vi "SW_Generate_SubCondition_text.vi"(8 "error in (no error)":errorcluster, 11 "Condition":T1 {"Response"."TTL pulse length, ms" min=0.0 max=10000.0 step=10.0 format="%0.0g"; "Specifier(s)"."Validity criteria(s)"."Validity value" min=0.0 step=0.1 format="%.2g"; "Specifier(s)"."Value" step=1.0 format="%#.2g"}) -> (0 "error out":errorcluster, 3 "SubCondition text":string[](array[string]))   [LabVIEW 2018, in "Tracker.lvlib"]
uses:
  Tracker.lvlib
  Controls/CTL_Conditions_Cluster.ctl
  Controls/CTL_Condition_type.ctl
  Controls/CTL_Comparison_type.ctl
  Controls/CTL_Validity_check_criteria.ctl
  Controls/CTL_Condition_response_type.ctl
panel:
  out "Array":string[](array[string])
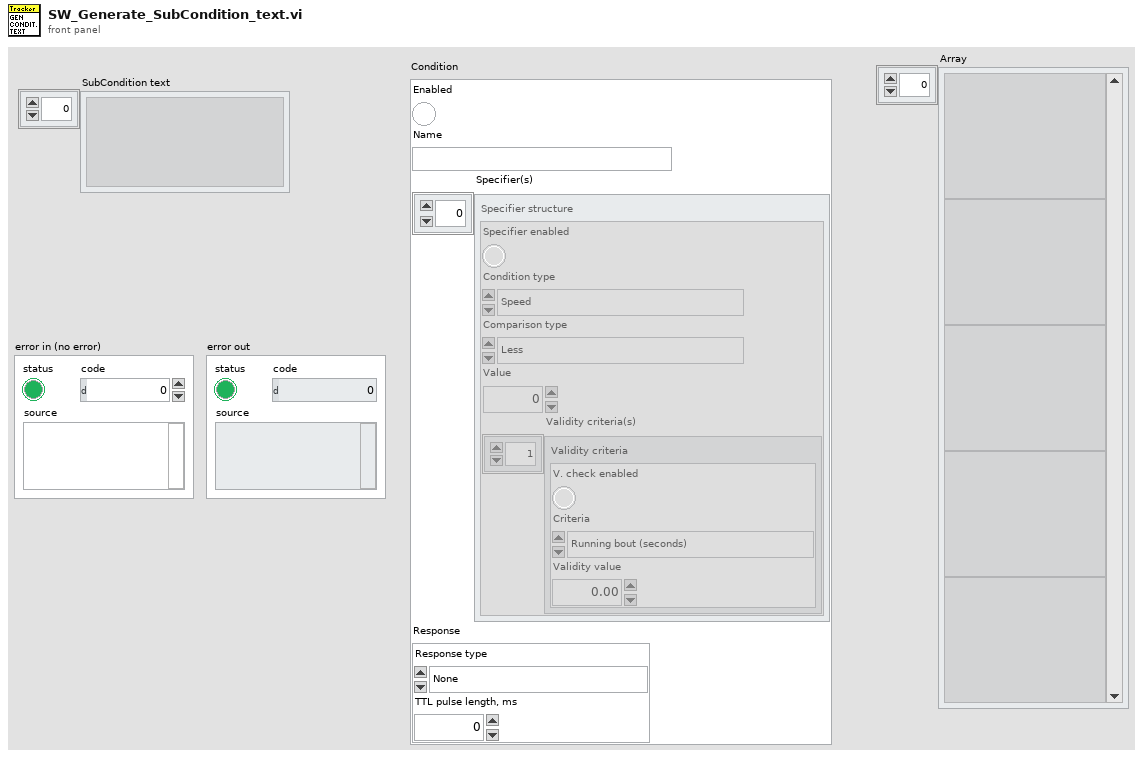
[diagram p1: front panel]
types:
  T1 = typedef "Tracker.lvlib/CTL_Conditions_Cluster.ctl" = cluster{"Enabled":bool, "Name":string, "Specifier(s)":cluster{"Specifier enabled":bool, "Condition type":T2, "Comparison type":T3, "Value":dbl, "Validity criteria(s)":cluster{"V. check enabled":bool, "Criteria":T4, "Validity value":dbl}[]}[], "Response":cluster{"Response type":T5, "TTL pulse length, ms":dbl}}
  T2 = typedef "Tracker.lvlib/CTL_Condition_type.ctl" = enum16{"Speed", "Zone", "Angle to wall"}
  T3 = typedef "Tracker.lvlib/CTL_Comparison_type.ctl" = enum16{"Less", "Less or Equal", "Equal", "Greater or Equal", "Greater", "Not Equal"}
  T4 = typedef "Tracker.lvlib/CTL_Validity_check_criteria.ctl" = enum16{"Running bout (seconds)", "Running bout (meters)"}
  T5 = typedef "Tracker.lvlib/CTL_Condition_response_type.ctl" = enum16{"None", "TTL"}
  T6 = cluster{"Specifier enabled":bool, "Condition type":T2, "Comparison type":T3, "Value":dbl, "Validity criteria(s)":cluster{"V. check enabled":bool, "Criteria":T4, "Validity value":dbl}[]}[]
  T7 = cluster{"V. check enabled":bool, "Criteria":T4, "Validity value":dbl}[]
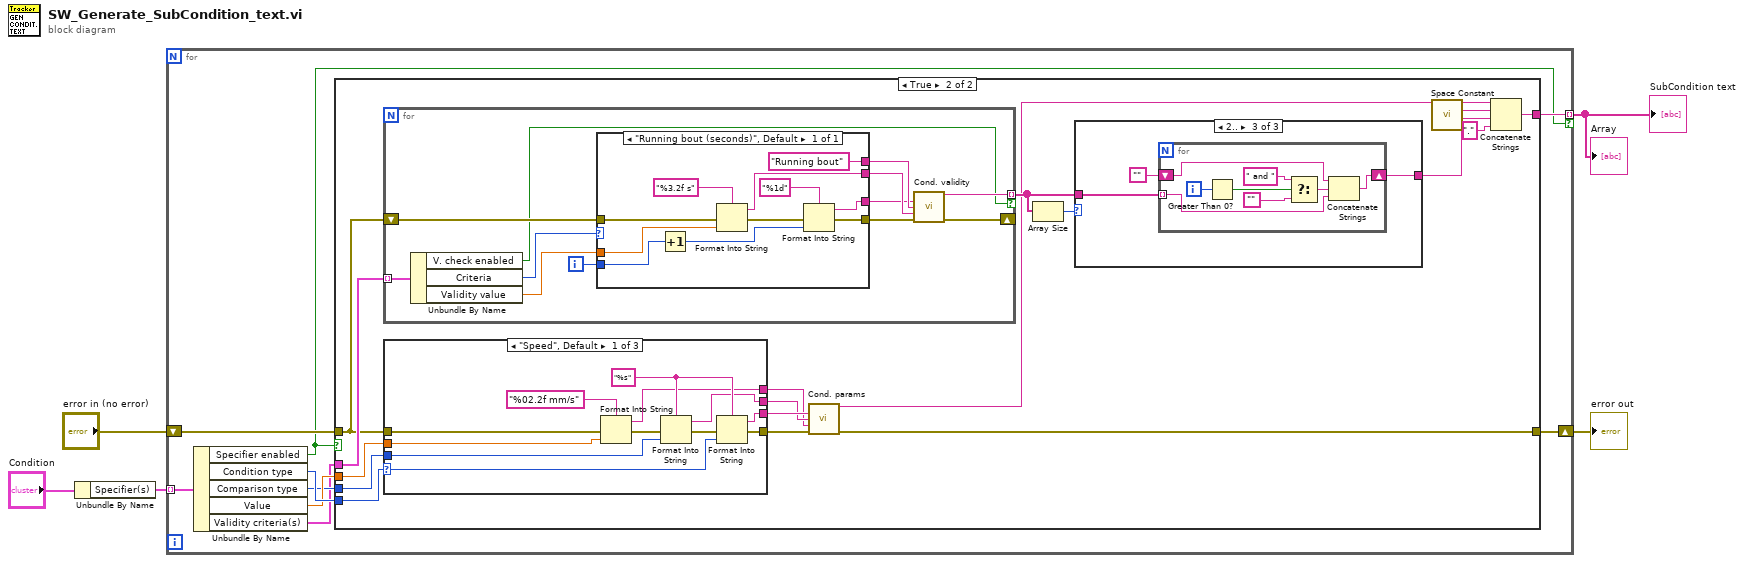
[diagram p0: block diagram]
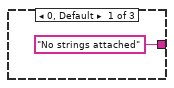
[diagram p3: hidden frame]
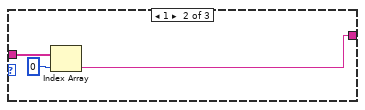
[diagram p4: hidden frame]
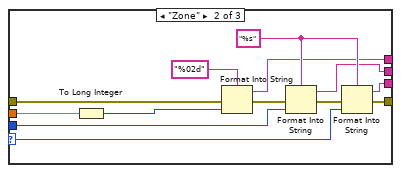
[diagram p5: hidden frame]
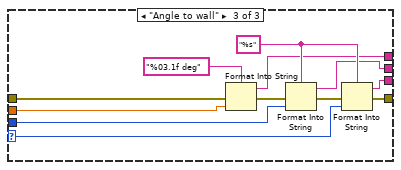
[diagram p6: hidden frame]
diagram:
  n1 = Unbundle By Name("Condition") -> ("Specifier(s)"=w4:T6)
  n2 = for {
    tunnel: w4 -> [w14] mode=indexing
    shift-right: [w9] -> w1
    shift-left: "error in (no error)" -> [w11]
    tunnel: [w8] -> w2 mode=indexing if=w7
    n3 = Unbundle By Name(w14) -> ("Specifier enabled"=w7:bool, "Condition type"=w13:T2, "Comparison type"=w10:T3, "Value"=w12:dbl, "Validity criteria(s)"=w6:T7)
    n4 = case shown="True" w7 {
      tunnel: w13 -> [_ w32]
      tunnel: w12 -> [_ w31]
      tunnel: w11 -> [w15 w23]
      tunnel: w10 -> [_ w30]
      tunnel: [w15 w25] -> w9
      tunnel: [_ w20] -> w8
      tunnel: w6 -> [_ w24]
      frame False {
      }
      frame True {
        n5 = for {
          tunnel: w24 -> [w59] mode=indexing
          shift-right: [w55] -> _
          shift-left: w23 -> [w57]
          tunnel: [w54] -> w21 mode=indexing if=w53
          i -> [w49]
          n6 = Unbundle By Name(w59) -> ("V. check enabled"=w53:bool, "Criteria"=w58:T4, "Validity value"=w56:dbl)
          n7 = case shown="\"Running bout (seconds)\", Default" w58 {
            tunnel: w57 -> [w68]
            tunnel: w56 -> [w69]
            tunnel: [w62] -> w52
            tunnel: ["Running bout"] -> w50
            tunnel: [w66] -> w51
            tunnel: w49 -> [w65]
            tunnel: [w61] -> w48
            frame "Running bout (seconds)", Default {
              n8 = Increment(x=w65) -> (x+1=w60:i32)
              n9 = Format Into String(format string="%3.2f s", error in=w68, w69) -> (resulting string=w66:string, error out=w63:errorcluster)  [unwired: 1 in]
              n10 = Format Into String(format string="%1d", error in=w63, w60) -> (resulting string=w61:string, error out=w62:errorcluster)  [unwired: 1 in]
            }
          }
          n11 = call "Cond. validity"("n"=w48, "param"=w50, "value"=w51, "error in (no error)"=w52) -> ("Result"=w54:string, "error out"=w55:errorcluster)  [unwired: 10 in]
        }
        n12 = case shown="\"Speed\", Default" w32 {
          selector: w32 -> [w80 w93 w106]
          tunnel: w31 -> [w81 w94 w100]
          tunnel: w23 -> [w78 w91 w104]
          tunnel: w30 -> [w79 w92 w105]
          tunnel: [w74 w83 w96] -> w29
          tunnel: [w73 w84 w97] -> w28
          tunnel: [w72 w85 w98] -> w27
          tunnel: [w71 w86 w99] -> w26
          frame "Speed", Default {
            w75 = "%s" ("format string")
            n13 = Format Into String(format string="%02.2f mm/s", error in=w78, w81) -> (resulting string=w72:string, error out=w77:errorcluster)  [unwired: 1 in]
            n14 = Format Into String(format string=w75, error in=w77, w79) -> (resulting string=w73:string, error out=w76:errorcluster)  [unwired: 1 in]
            n15 = Format Into String(format string=w75, error in=w76, w80) -> (resulting string=w74:string, error out=w71:errorcluster)  [unwired: 1 in]
          }
          frame "Zone" {
            w88 = "%s" ("format string")
            n16 = To Long Integer(number=w94) -> (32bit integer=w87:i32)
            n17 = Format Into String(format string="%02d", error in=w91, w87) -> (resulting string=w85:string, error out=w90:errorcluster)  [unwired: 1 in]
            n18 = Format Into String(format string=w88, error in=w90, w92) -> (resulting string=w84:string, error out=w89:errorcluster)  [unwired: 1 in]
            n19 = Format Into String(format string=w88, error in=w89, w93) -> (resulting string=w83:string, error out=w86:errorcluster)  [unwired: 1 in]
          }
          frame "Angle to wall" {
            w101 = "%s" ("format string")
            n20 = Format Into String(format string="%03.1f deg", error in=w104, w100) -> (resulting string=w98:string, error out=w103:errorcluster)  [unwired: 1 in]
            n21 = Format Into String(format string=w101, error in=w103, w105) -> (resulting string=w97:string, error out=w102:errorcluster)  [unwired: 1 in]
            n22 = Format Into String(format string=w101, error in=w102, w106) -> (resulting string=w96:string, error out=w99:errorcluster)  [unwired: 1 in]
          }
        }
        n23 = call "Cond. params"("condname"=w29, "comptype"=w28, "comvalue"=w27, "error in (no error)"=w26) -> ("Result"=w17:string, "error out"=w25:errorcluster)  [unwired: 10 in]
        n24 = Array Size(array=w21) -> (size(s)=w22:i32)
        n25 = case shown="2.." w22 {
          tunnel: w21 -> [_ w36 w39]
          tunnel: ["No strings attached" ("Result") w34 w37] -> w16
          frame 0, Default {
          }
          frame 1 {
            n26 = Index Array(array=w36, index=0) -> (element=w34:string)
          }
          frame 2.. {
            n27 = for {
              shift-right: [w46] -> w37
              shift-left: "" -> [w47]
              tunnel: w39 -> [w40] mode=indexing
              i -> [w45]
              n28 = Greater Than 0?(x=w45) -> (x > 0?=w44:bool)
              n29 = Select(t=" and ", s=w44, f="") -> (s? t:f=w41:string)
              n30 = Concatenate Strings(w47, w41, w40) -> (w46:string)
            }
          }
        }
        n31 = call <vilib>:"Space Constant.vi"() -> ("String"=w19:string)
        n32 = Concatenate Strings(w17, w19, w16, "." ("string")) -> (w20:string)
      }
    }
  }
  "error out" <- w1
  "SubCondition text" <- w2
  "Array" <- w2
